vi "Create Caption Object.vi"(8 "error in (no error)":errorcluster, 9 "Label Width":T1, 10 "3D Plot.lvclass in":refnum<class "3D Plot.lvclass">, 11 "Axis Object In":refnum<vi>) -> (0 "error out":errorcluster, 2 "3D Plot.lvclass out":refnum<class "3D Plot.lvclass">, 3 "Axis Object Out":refnum<vi>)   [LabVIEW 2017, in "3D Plot.lvclass"]
uses:
  <vilib>/Math Plots/3D Math Plots/3D Plot/3D Plot/3D Plot.lvclass
  <vilib>/Math Plots/3D Math Plots/3D Plot/3D Plot/Typedef/Label Width.ctl
  <vilib>/Math Plots/3D Math Plots/3D Plot/3D Plot/3D Plot.lvclass/3D Plot.ctl
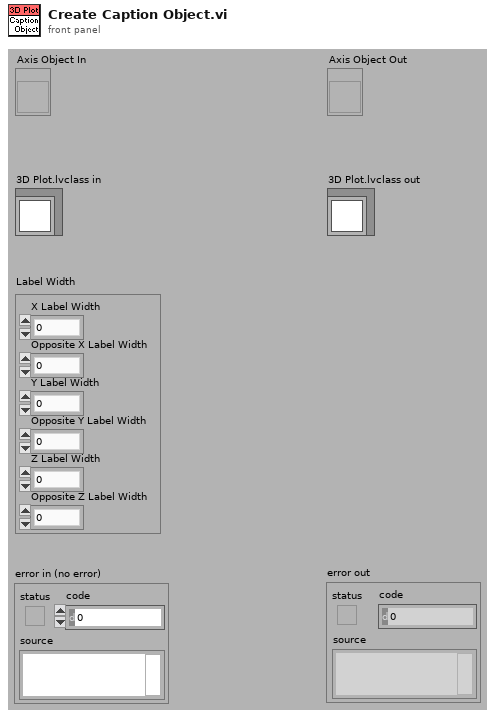
[diagram p1: front panel]
types:
  T1 = typedef "3D Plot.lvclass/Label Width.ctl" = cluster{"X Label Width":sgl, "Opposite X Label Width":sgl, "Y Label Width":sgl, "Opposite Y Label Width":sgl, "Z Label Width":sgl, "Opposite Z Label Width":sgl}
  T2 = enum16{"X", "Y", "Z", "X Opposite", "Y Opposite", "Z Opposite"}
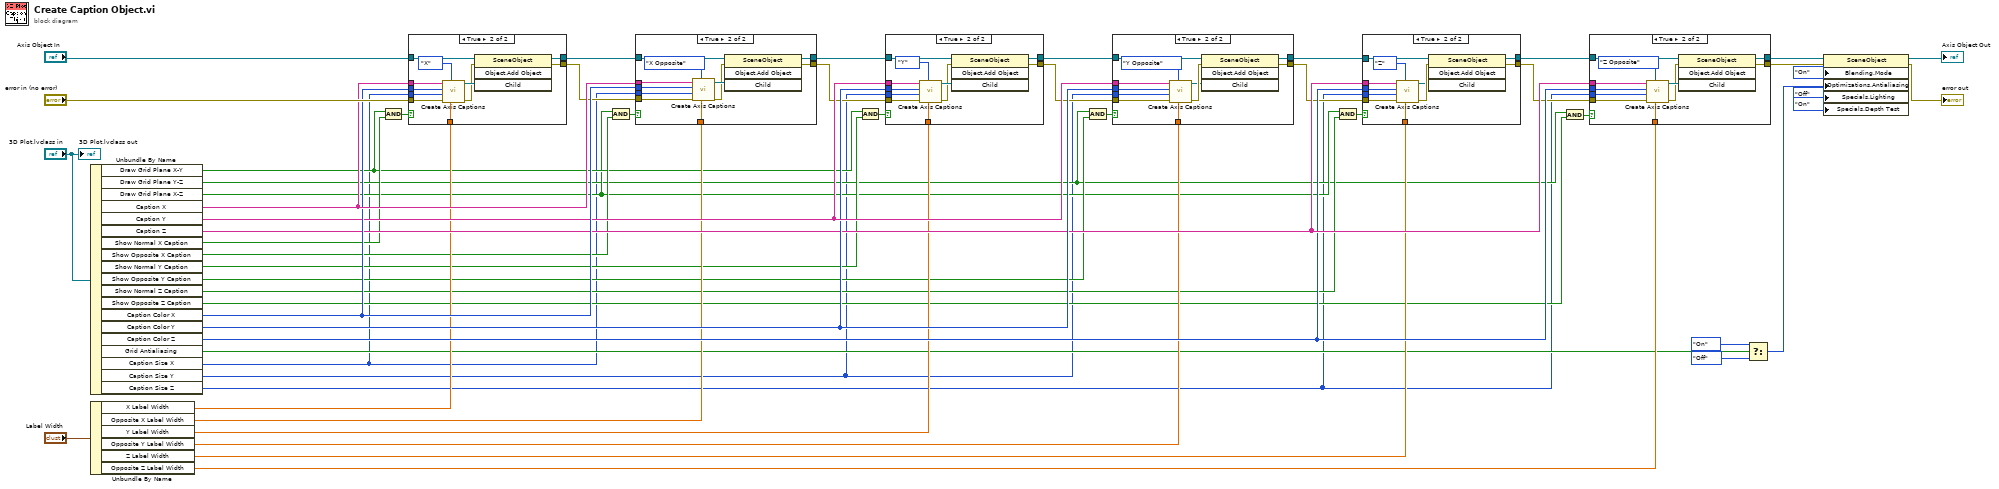
[diagram p0: block diagram]
diagram:
  n1 = Unbundle By Name("3D Plot.lvclass in") -> ("Draw Grid Plane X-Y"=w24:bool, "Draw Grid Plane Y-Z"=w14:bool, "Draw Grid Plane X-Z"=w17:bool, "Caption X"=w49:string, "Caption Y"=w46:string, "Caption Z"=w43:string, "Show Normal X Caption"=w28:bool, "Show Opposite X Caption"=w26:bool, "Show Normal Y Caption"=w23:bool, "Show Opposite Y Caption"=w21:bool, "Show Normal Z Caption"=w19:bool, "Show Opposite Z Caption"=w15:bool, "Caption Color X"=w48:u32, "Caption Color Y"=w45:u32, "Caption Color Z"=w42:u32, "Grid Antialiasing"=w5:bool, "Caption Size X"=w3:u16, "Caption Size Y"=w1:u16, "Caption Size Z"=w2:u16)
  n2 = Unbundle By Name("Label Width") -> ("X Label Width"=w29:sgl, "Opposite X Label Width"=w30:sgl, "Y Label Width"=w32:sgl, "Opposite Y Label Width"=w31:sgl, "Z Label Width"=w39:sgl, "Opposite Z Label Width"=w38:sgl)
  n3 = And(x=w24, y=w28) -> (x .and. y?=w27:bool)
  n4 = case shown="True" w27 {
    tunnel: [w57 w68] -> w50
    tunnel: "Axis Object In" -> [w57 w66]
    tunnel: w29 -> [_ w58]
    tunnel: w3 -> [_ w67]
    tunnel: w49 -> [_ w62]
    tunnel: w48 -> [_ w61]
    tunnel: "error in (no error)" -> [w56 w60]
    tunnel: [w56 w63] -> w37
    frame False {
    }
    frame True {
      n5 = call <vilib>:"Create Axis Captions.vi"("Label Width"=w58, "Which Axis?"=T2."X", "error in (no error)"=w60, "Caption Size"=w67, "Caption Color"=w61, "Caption Text"=w62) -> ("error out"=w64:errorcluster, "New Caption Object"=w65:refnum<vi>)  [unwired: 1 in, 3 out]
      n6 = invoke class="SceneObject" method="Object.Add Object"(reference=w66, error in=w64, "Child"=w65) -> (reference out=w68:refnum<vi>, error out=w63:errorcluster)  [unwired: 1 in, 2 out]
    }
  }
  n7 = And(x=w17, y=w26) -> (x .and. y?=w25:bool)
  n8 = case shown="True" w25 {
    tunnel: [w70 w81] -> w47
    tunnel: w50 -> [w70 w80]
    tunnel: w30 -> [_ w71]
    tunnel: w3 -> [_ w75]
    tunnel: w49 -> [_ w78]
    tunnel: w48 -> [_ w77]
    tunnel: w37 -> [w69 w76]
    tunnel: [w69 w79] -> w36
    frame False {
    }
    frame True {
      n9 = call <vilib>:"Create Axis Captions.vi"("Label Width"=w71, "Which Axis?"=T2."X Opposite", "error in (no error)"=w76, "Caption Size"=w75, "Caption Color"=w77, "Caption Text"=w78) -> ("error out"=w72:errorcluster, "New Caption Object"=w73:refnum<vi>)  [unwired: 1 in, 3 out]
      n10 = invoke class="SceneObject" method="Object.Add Object"(reference=w80, error in=w72, "Child"=w73) -> (reference out=w81:refnum<vi>, error out=w79:errorcluster)  [unwired: 1 in, 2 out]
    }
  }
  n11 = And(x=w24, y=w23) -> (x .and. y?=w22:bool)
  n12 = case shown="True" w22 {
    tunnel: [w83 w94] -> w44
    tunnel: w47 -> [w83 w93]
    tunnel: w32 -> [_ w84]
    tunnel: w1 -> [_ w88]
    tunnel: w46 -> [_ w91]
    tunnel: w45 -> [_ w90]
    tunnel: w36 -> [w82 w89]
    tunnel: [w82 w92] -> w35
    frame False {
    }
    frame True {
      n13 = call <vilib>:"Create Axis Captions.vi"("Label Width"=w84, "Which Axis?"=T2."Y", "error in (no error)"=w89, "Caption Size"=w88, "Caption Color"=w90, "Caption Text"=w91) -> ("error out"=w86:errorcluster, "New Caption Object"=w87:refnum<vi>)  [unwired: 1 in, 3 out]
      n14 = invoke class="SceneObject" method="Object.Add Object"(reference=w93, error in=w86, "Child"=w87) -> (reference out=w94:refnum<vi>, error out=w92:errorcluster)  [unwired: 1 in, 2 out]
    }
  }
  n15 = And(x=w14, y=w21) -> (x .and. y?=w20:bool)
  n16 = case shown="True" w20 {
    tunnel: [w96 w107] -> w41
    tunnel: w44 -> [w96 w106]
    tunnel: w31 -> [_ w97]
    tunnel: w1 -> [_ w101]
    tunnel: w46 -> [_ w104]
    tunnel: w45 -> [_ w103]
    tunnel: w35 -> [w95 w102]
    tunnel: [w95 w105] -> w34
    frame False {
    }
    frame True {
      n17 = call <vilib>:"Create Axis Captions.vi"("Label Width"=w97, "Which Axis?"=T2."Y Opposite", "error in (no error)"=w102, "Caption Size"=w101, "Caption Color"=w103, "Caption Text"=w104) -> ("error out"=w100:errorcluster, "New Caption Object"=w99:refnum<vi>)  [unwired: 1 in, 3 out]
      n18 = invoke class="SceneObject" method="Object.Add Object"(reference=w106, error in=w100, "Child"=w99) -> (reference out=w107:refnum<vi>, error out=w105:errorcluster)  [unwired: 1 in, 2 out]
    }
  }
  n19 = And(x=w17, y=w19) -> (x .and. y?=w18:bool)
  n20 = case shown="True" w18 {
    tunnel: [w109 w120] -> w40
    tunnel: w41 -> [w109 w119]
    tunnel: w39 -> [_ w110]
    tunnel: w2 -> [_ w114]
    tunnel: w43 -> [_ w117]
    tunnel: w42 -> [_ w116]
    tunnel: w34 -> [w108 w113]
    tunnel: [w108 w118] -> w33
    frame False {
    }
    frame True {
      n21 = call <vilib>:"Create Axis Captions.vi"("Label Width"=w110, "Which Axis?"=T2."Z", "error in (no error)"=w113, "Caption Size"=w114, "Caption Color"=w116, "Caption Text"=w117) -> ("error out"=w112:errorcluster, "New Caption Object"=w111:refnum<vi>)  [unwired: 1 in, 3 out]
      n22 = invoke class="SceneObject" method="Object.Add Object"(reference=w119, error in=w112, "Child"=w111) -> (reference out=w120:refnum<vi>, error out=w118:errorcluster)  [unwired: 1 in, 2 out]
    }
  }
  n23 = And(x=w14, y=w15) -> (x .and. y?=w16:bool)
  n24 = case shown="True" w16 {
    tunnel: [w122 w133] -> w8
    tunnel: w40 -> [w122 w132]
    tunnel: w38 -> [_ w123]
    tunnel: w2 -> [_ w127]
    tunnel: w43 -> [_ w130]
    tunnel: w42 -> [_ w129]
    tunnel: w33 -> [w121 w128]
    tunnel: [w121 w131] -> w7
    frame False {
    }
    frame True {
      n25 = call <vilib>:"Create Axis Captions.vi"("Label Width"=w123, "Which Axis?"=T2."Z Opposite", "error in (no error)"=w128, "Caption Size"=w127, "Caption Color"=w129, "Caption Text"=w130) -> ("error out"=w124:errorcluster, "New Caption Object"=w125:refnum<vi>)  [unwired: 1 in, 3 out]
      n26 = invoke class="SceneObject" method="Object.Add Object"(reference=w132, error in=w124, "Child"=w125) -> (reference out=w133:refnum<vi>, error out=w131:errorcluster)  [unwired: 1 in, 2 out]
    }
  }
  n27 = Select(t=enum16{"Inherit Value", "Off", "On"}."On" ("Optimizations:Antialiasing"), s=w5, f=enum16{"Inherit Value", "Off", "On"}."Off" ("Optimizations:Antialiasing")) -> (s? t:f=w6:enum16{"Inherit Value", "Off", "On"})
  n28 = property class="SceneObject"(reference=w8, error in=w7, "Blending.Mode"=enum16{"Inherit Value", "Off", "On"}."On" ("Specials:Lighting"), "Optimizations.Antialiasing"=w6, "Specials.Lighting"=enum16{"Inherit Value", "Off", "On"}."Off" ("Blending:Mode"), "Specials.Depth Test"=enum16{"Inherit Value", "Off", "On"}."On" ("Specials:Depth Test")) -> (reference out=→"Axis Object Out":refnum<vi>, error out=→"error out":errorcluster)
  "3D Plot.lvclass out" <- "3D Plot.lvclass in"
